vi "Transfer image from RT to FPGA (SubVI).vi"(8 "Timeout":i32, 9 "Image Size in":T2={"Rows (X)"=256, "Colums (Y)"=256}, 10 "Image Pixels (U8)":u8[][](array[numeric]), 11 "FPGA Refnum in":T1) -> (1 "Image Size out":T2={"Rows (X)"=256, "Colums (Y)"=256}, 3 "FPGA Refnum out":T1)   [LabVIEW 2025, in "SoC IP Library.lvlib"]
uses:
  SoC IP Library.lvlib
  Controls/Image Size.ctl
  Controls/FPGA Reference Type.ctl
  <vilib>/Utility/error.llb/Error Cluster From Error Code.vi
  <vilib>/rvi/errors/niLvFpgaAdjustHostInterfaceError.vi
  <vilib>/rvi/interface/nirviMethod/nirviMethod.xnode
  <vilib>/FPGAPlugInAG/Dynamic/niLvFpga_WriteFifo_Dynamic.vi
  <vilib>/rvi/errors/niLvFpgaMergeErrorWithErrorCode.vi
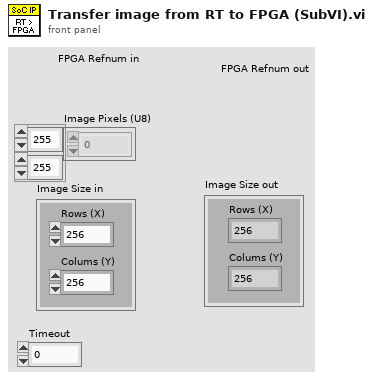
[diagram p1: front panel]
types:
  T1 = typedef "SoC IP Library.lvlib/FPGA Reference Type.ctl" = refnum<k20>
  T2 = typedef "SoC IP Library.lvlib/Image Size.ctl" = cluster{"Rows (X)":u16, "Colums (Y)":u16}
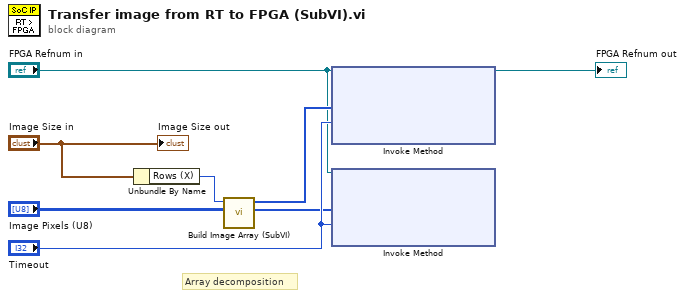
[diagram p0: block diagram]
diagram:
  # "Array decomposition"
  n1 = Unbundle By Name("Image Size in") -> ("Rows (X)"=w4:u16)
  n2 = call "Build Image Array (SubVI).vi"("Image Pixels (U8) in"="Image Pixels (U8)", "Rows (X)"=w4) -> ("Image Pixels B (U8) 3"=w5:u8[], "Image Pixels A (U8) out"=w6:u8[])  [unwired: 8 in]
  n3 = xnode "Invoke Method"("FPGA VI Reference In"="FPGA Refnum in", "Data"=w6, "Timeout (ms)"="Timeout") -> ("FPGA VI Reference Out"=→"FPGA Refnum out":T1)  [unwired: 1 in, 2 out]
  n4 = xnode "Invoke Method"("FPGA VI Reference In"="FPGA Refnum in", "Data"=w5, "Timeout (ms)"="Timeout") -> ()  [unwired: 1 in, 3 out]
  "Image Size out" <- "Image Size in"
